vi "test-TimeInterpRotation-Test2.vi"() -> (3 "All tests passed":bool)   [LabVIEW 2019]
uses:
  <vilib>/Rock Robotics/WPI/ThirdParty/JAS_Junk/TrajLib/TimeInterpRotation2d_CleanUp.vi
  <vilib>/Rock Robotics/WPI/ThirdParty/JAS_Junk/TrajLib/MathUtil_InputModulus.vi
  <vilib>/gmath/interp.llb/Search Ordered Table.vi
  <vilib>/Rock Robotics/WPI/ThirdParty/JAS_Junk/TrajLib/Trajectory_Library.lvlib
panel:
  out "Add Error":bool
  out "Error 1":bool
  out "Error 2":bool
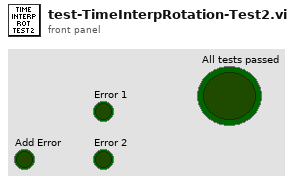
[diagram p1: front panel]
types:
  T1 = typedef "Trajectory_Library.lvlib/TIME_INTERPOLATABLE_ROTATION.ctl" = cluster{"TimeStamps":dbl[], "RotationValues":T2[], "Min_TimeStamp":dbl, "Max_TimeStamp":dbl, "ItemCount":i32, "MaxBufferTime":dbl}
  T2 = typedef "Trajectory_Library.lvlib/ROTATION2D.ctl" = cluster{"VALUE":dbl, "COS":dbl, "SIN":dbl}
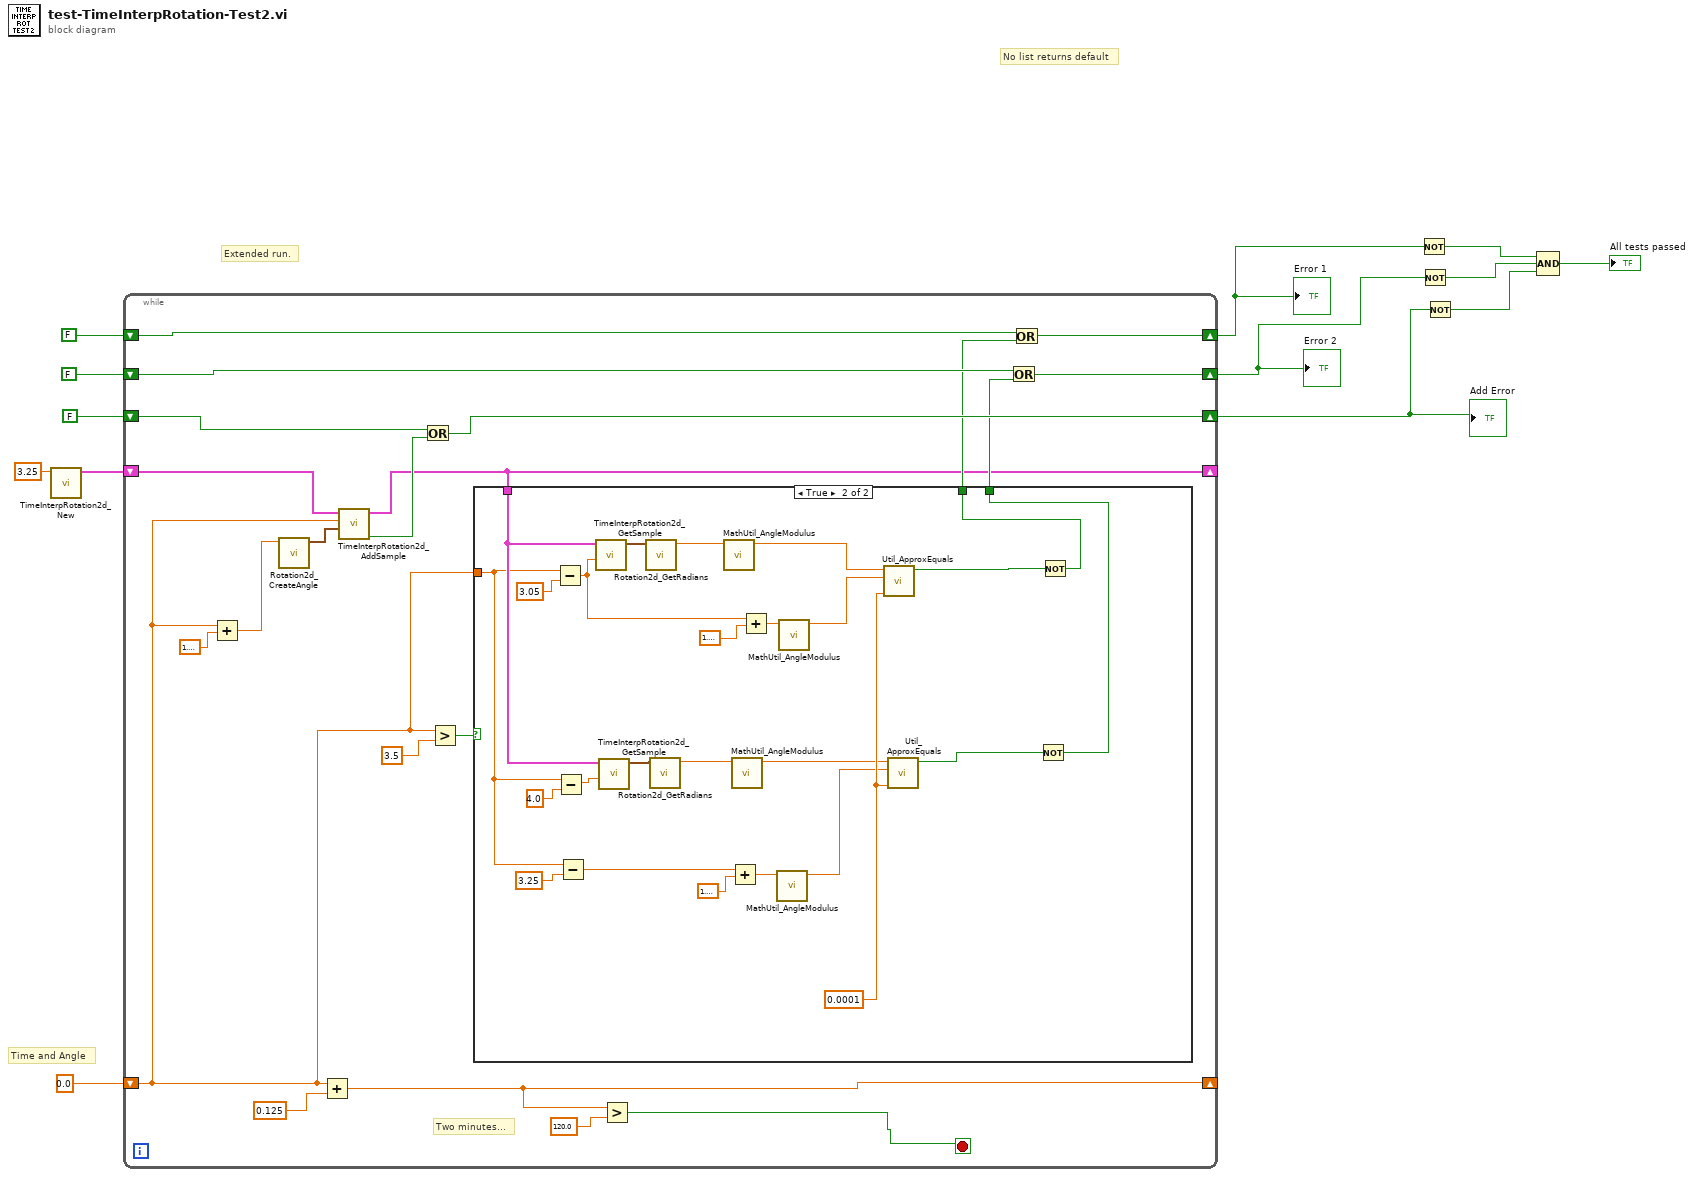
[diagram p0: block diagram]
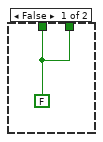
[diagram p2: hidden frame]
diagram:
  # "Extended run."
  # "Time and Angle"
  # "No list returns default"
  n1 = call <vilib>:"TimeInterpRotation2d_New.vi"("MaxTime"=3.25) -> ("TimeInterpRotation"=w11:T1)  [unwired: 10 in]
  n2 = while {
    shift-right: [w31] -> _
    shift-left: 0.0 -> [w23]
    shift-right: [w15] -> _
    shift-left: w11 -> [w29]
    shift-right: [w20] -> w7
    shift-left: FALSE -> [w26]
    shift-right: [w21] -> w5
    shift-left: FALSE -> [w18]
    shift-right: [w22] -> w6
    shift-left: FALSE -> [w19]
    stop <- w34 stop-if-true
    # "Two minutes..."
    n3 = Add(x=w23, y=1.5707963267948966) -> (x+y=w14:dbl)
    n4 = call <vilib>:"Rotation2d_CreateAngle.vi"("Angle"=w14) -> ("ROTATION"=w30:T2)  [unwired: 10 in]
    n5 = Add(x=w23, y=0.125) -> (x+y=w31:dbl)
    n6 = call <vilib>:"TimeInterpRotation2d_AddSample.vi"("RotationValue"=w30, "TimeStamp"=w23, "in TimeInterpRotation"=w29) -> ("Error"=w27:bool, "out TimeInterpRotation"=w15:T1)  [unwired: 7 in]
    n7 = Or(x=w26, y=w27) -> (x .or. y?=w20:bool)
    n8 = Greater?(x=w23, y=3.5) -> (0:w25:bool)
    n9 = case shown="True" w25 {
      tunnel: w15 -> [_ w60]
      tunnel: w23 -> [_ w53]
      tunnel: [w35 w42] -> w17
      tunnel: [w35 w41] -> w16
      frame False {
        w35 = FALSE
      }
      frame True {
        w47 = 0.0001 ("Tolerance")
        n10 = Subtract(x=w53, y=3.05) -> (x-y=w46:dbl)
        n11 = Subtract(x=w53, y=4.0) -> (x-y=w58:dbl)
        n12 = Subtract(x=w53, y=3.25) -> (x-y=w51:dbl)
        n13 = call <vilib>:"TimeInterpRotation2d_GetSample.vi"("TimeStamp"=w46, "TimeInterpRotation"=w60) -> ("OutputRotation"=w56:T2)  [unwired: 9 in]
        n14 = call <vilib>:"TimeInterpRotation2d_GetSample.vi"("TimeStamp"=w58, "TimeInterpRotation"=w60) -> ("OutputRotation"=w38:T2)  [unwired: 9 in]
        n15 = call <vilib>:"Rotation2d_GetRadians.vi"("in ROTATION"=w56) -> ("AngleRadians"=w40:dbl)  [unwired: 10 in]
        n16 = call <vilib>:"Rotation2d_GetRadians.vi"("in ROTATION"=w38) -> ("AngleRadians"=w37:dbl)  [unwired: 10 in]
        n17 = call <vilib>:"MathUtil_AngleModulus.vi"("InputAngle"=w40) -> ("ModulsAngle"=w43:dbl)  [unwired: 10 in]
        n18 = Add(x=w51, y=1.5707963267948966) -> (x+y=w49:dbl)
        n19 = call <vilib>:"MathUtil_AngleModulus.vi"("InputAngle"=w37) -> ("ModulsAngle"=w44:dbl)  [unwired: 10 in]
        n20 = Add(x=w46, y=1.5707963267948966) -> (x+y=w50:dbl)
        n21 = call <vilib>:"MathUtil_AngleModulus.vi"("InputAngle"=w49) -> ("ModulsAngle"=w45:dbl)  [unwired: 10 in]
        n22 = call <vilib>:"MathUtil_AngleModulus.vi"("InputAngle"=w50) -> ("ModulsAngle"=w48:dbl)  [unwired: 10 in]
        n23 = call <vilib>:"Util_ApproxEquals.vi"("Tolerance"=w47, "Value 2"=w48, "Value 1"=w43) -> ("ApproxEquals"=w39:bool)  [unwired: 8 in]
        n24 = call <vilib>:"Util_ApproxEquals.vi"("Tolerance"=w47, "Value 2"=w45, "Value 1"=w44) -> ("ApproxEquals"=w36:bool)  [unwired: 8 in]
        n25 = Not(x=w36) -> (.not. x?=w41:bool)
        n26 = Not(x=w39) -> (.not. x?=w42:bool)
      }
    }
    n27 = Greater?(x=w31, y=120.0) -> (0:w34:bool)
    n28 = Or(x=w18, y=w16) -> (x .or. y?=w21:bool)
    n29 = Or(x=w19, y=w17) -> (x .or. y?=w22:bool)
  }
  "Add Error" <- w7
  "Error 1" <- w6
  "Error 2" <- w5
  n30 = Not(x=w6) -> (.not. x?=w4:bool)
  n31 = Not(x=w5) -> (.not. x?=w3:bool)
  n32 = Not(x=w7) -> (.not. x?=w2:bool)
  n33 = Compound Arithmetic op=AND(w4, w3, w2) -> (→"All tests passed":bool)
